vi "Wait for zero.vi"(4 "exit button ref":refnum<vi>, 5 "Starting angle M1":dbl, 6 "stop motors ref":refnum<vi>, 7 "Starting angle M2":dbl, 8 "error in (no error)":errorcluster, 9 "Home ctrl ref":refnum<vi>, 10 "Move motor ctrl ref":refnum<vi>, 11 "VISA resource name":refnum<visa-resource-name>) -> (0 "error out":errorcluster)   [LabVIEW 2025]
uses:
  Public/Controls/Move motor parameters--cluster.ctl
  Public/Controls/Motor direction.ctl
  Public/Controls/Step style.ctl
  Public/Write--move.vi
  Control de MaP.lvlib
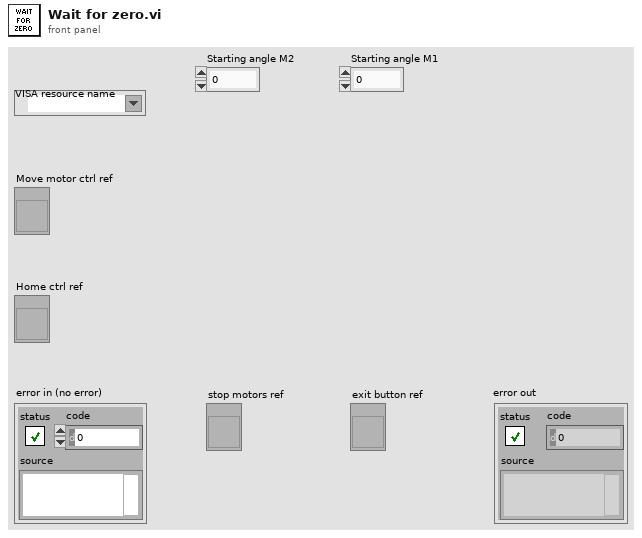
[diagram p1: front panel]
types:
  T1 = typedef "Control de MaP.lvlib/Move motor parameters--cluster.ctl" = cluster{"Action":u8, "Direction motor 1":T2, "Direction motor 2":T2, "Steps motor 1":u16, "Steps motor 2":u16, "Step style motor 1":T3, "Step style motor 2":T3}
  T2 = typedef "Control de MaP.lvlib/Motor direction.ctl" = u8
  T3 = typedef "Control de MaP.lvlib/Step style.ctl" = u8
  T4 = enum8{"Enabled", "Disabled", "Disabled and Grayed Out"}
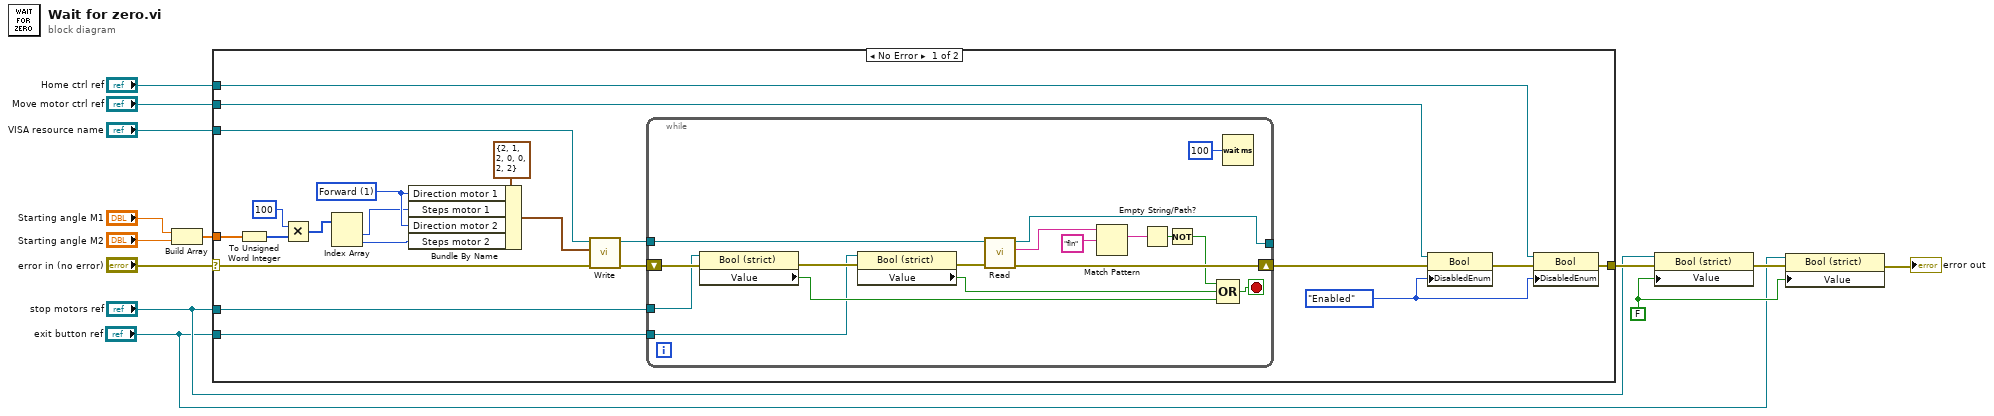
[diagram p0: block diagram]
diagram:
  w2 = FALSE ("Value")
  n1 = Build Array("Starting angle M1", "Starting angle M2") -> (w9:dbl[])
  n2 = case shown="No Error" "error in (no error)" {
    selector: "error in (no error)" -> [w31 w52]
    tunnel: "VISA resource name" -> [w32 _]
    tunnel: w9 -> [w27 _]
    tunnel: [w18 w52] -> w6
    tunnel: "Move motor ctrl ref" -> [w20 _]
    tunnel: "Home ctrl ref" -> [w17 _]
    tunnel: "stop motors ref" -> [w15 _]
    tunnel: "exit button ref" -> [w14 _]
    frame No Error {
      w16 = T4."Enabled" ("f")
      w30 = T2 1 items=["", "Forward", "Backward"] ("Direction motor 1")
      n3 = To Unsigned Word Integer(number=w27) -> (unsigned 16bit integer=w29:u16[])
      n4 = Multiply(x=u16 100 ("y"), y=w29) -> (x*y=w26:u16[])
      n5 = Index Array(array=w26) -> (element #1=w25:u16, element #2=w24:u16)  [unwired: 2 in]
      n6 = Bundle By Name(cluster=T1 {"Action"=2, "Direction motor 1"=1, "Direction motor 2"=2, "Steps motor 1"=0, "Steps motor 2"=0, "Step style motor 1"=2, "Step style motor 2"=2} ("Comando"), "Direction motor 1"=w30, "Steps motor 1"=w25, "Direction motor 2"=w30, "Steps motor 2"=w24) -> (w34:T1)
      n7 = call-poly "Write.vi"("error in (no error)"=w31, "Comando"=w34, "VISA resource name"=w32) -> ("error out"=w23:errorcluster, "VISA resource name out"=w22:refnum<visa-resource-name>)  [unwired: 6 in, 1 out]
      n8 = while {
        shift-right: [w51] -> w21
        shift-left: w23 -> [w42]
        tunnel: w22 -> [w50]
        tunnel: [w44] -> _
        tunnel: w15 -> [w41]
        tunnel: w14 -> [w35]
        stop <- w40 stop-if-true
        n9 = property class="Bool (strict)"(reference=w41, error in=w42) -> (error out=w38:errorcluster, "Value"=w39:bool)  [unwired: 1 out]
        n10 = property class="Bool (strict)"(reference=w35, error in=w38) -> (error out=w37:errorcluster, "Value"=w36:bool)  [unwired: 1 out]
        n11 = call "Read.vi"("error in (no error)"=w37, "VISA resource name"=w50) -> ("error out"=w51:errorcluster, "Recibo de Datos"=w46:string, "VISA resource name out"=w44:refnum<visa-resource-name>)  [unwired: 6 in, 1 out]
        n12 = Match Pattern(string=w46, regular expression="fin") -> (match substring=w48:string)  [unwired: 1 in, 3 out]
        n13 = Empty String/Path?(string/path=w48) -> (empty?=w47:bool)
        n14 = Not(x=w47) -> (.not. x?=w45:bool)
        n15 = Compound Arithmetic op=OR(w45, w36, w39) -> (w40:bool)
        n16 = Wait (ms)(milliseconds to wait=u32 100) -> ()  [unwired: 1 out]
      }
      n17 = property on="Property Node" class="Bool"(reference=w20, error in=w21, "DisabledEnum"=w16) -> (error out=w19:errorcluster)  [unwired: 1 out]
      n18 = property on="Property Node" class="Bool"(reference=w17, error in=w19, "DisabledEnum"=w16) -> (error out=w18:errorcluster)  [unwired: 1 out]
    }
    frame Error {
    }
  }
  n19 = property class="Bool (strict)"(reference="stop motors ref", error in=w6, "Value"=w2) -> (error out=w4:errorcluster)  [unwired: 1 out]
  n20 = property class="Bool (strict)"(reference="exit button ref", error in=w4, "Value"=w2) -> (error out=→"error out":errorcluster)  [unwired: 1 out]
